vi "Accel Values View.vi"() -> ()   [LabVIEW 2016, in "M1M3SupportEUI_Views.lvlib"]
uses:
  M1M3SupportEUI_Views.lvlib
  Model/Model.lvclass
panel:
  in  "Model in":refnum<class "Model.lvclass">
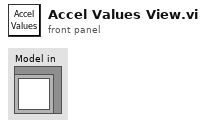
[diagram p1: front panel]
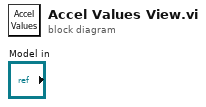
[diagram p0: block diagram]
diagram:
